vi "Test_EndOfList_ReturnLastItem.vi"(8 "error in (no error)":errorcluster, 11 "TestCase in":refnum<class "TestStringList.lvclass">) -> (0 "error out":errorcluster, 3 "TestCase out":refnum<class "TestStringList.lvclass">)   [LabVIEW 2015, in "StringList.lvlib" / "TestStringList.lvclass"]
uses:
  TestStringList.lvclass
  <vilib>/addons/_JKI Toolkits/VI Tester/TestCase.llb/TestCase.lvclass
  StringList.lvclass
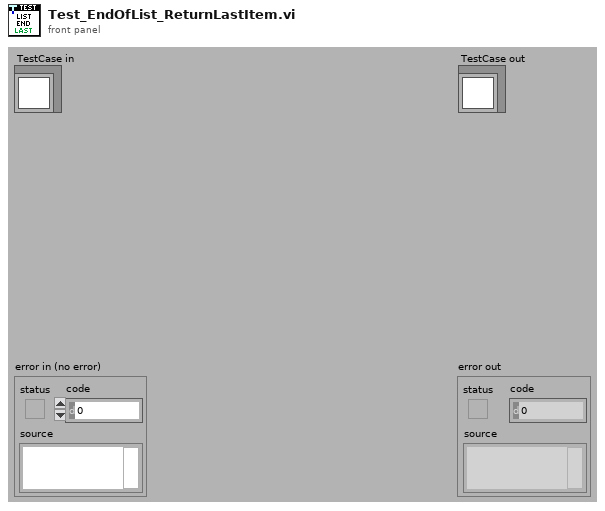
[diagram p1: front panel]
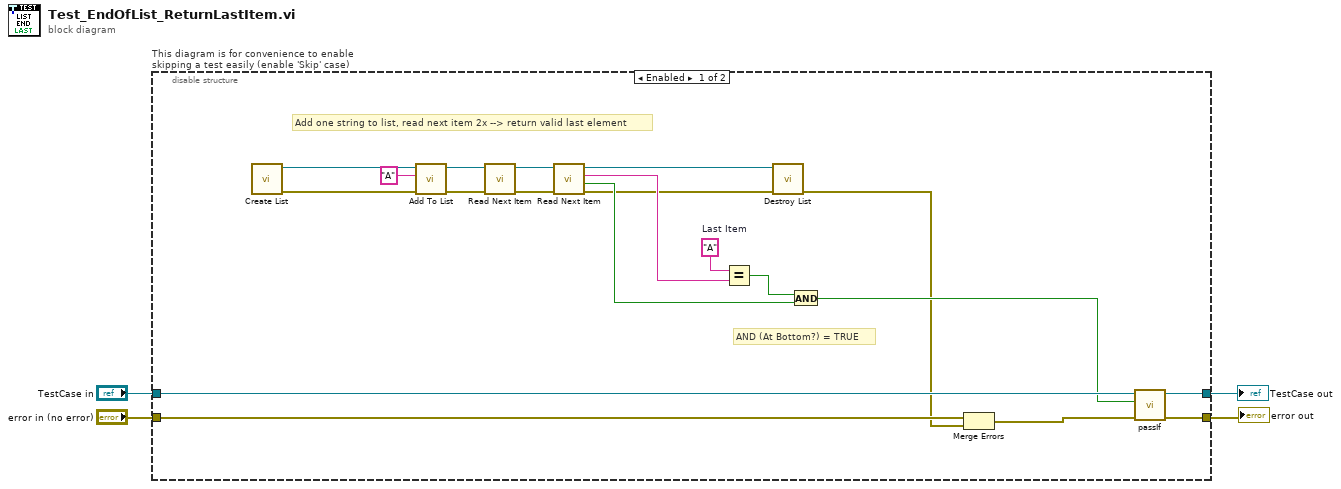
[diagram p0: block diagram]
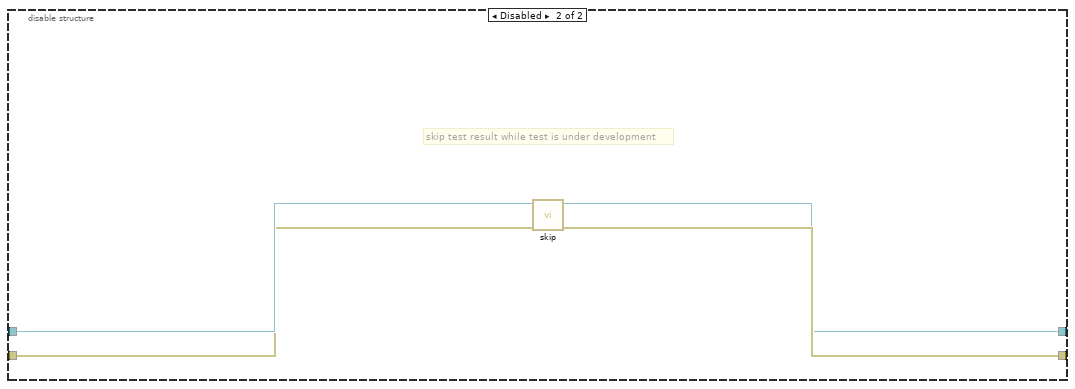
[diagram p2: hidden frame]
diagram:
  n1 = disable-structure "This diagram is for convenience to enable skipping a test easily (enable 'Skip' case)" shown="Enabled" {
    disable-tunnel: "TestCase in" -> [w24 w28]
    disable-tunnel: [w23 w26] -> w1
    disable-tunnel: [w22 w27] -> w3
    disable-tunnel: "error in (no error)" -> [w21 w25]
    frame Enabled {
      w15 = "A"  # Last Item
      # "AND (At Bottom?) = TRUE"
      # "Add one string to list, read next item 2x --> return valid last element"
      n2 = call "Create List.vi"() -> ("error out"=w10:errorcluster, "StringList Reference"=w17:refnum<data-value>)  [unwired: 10 in]
      n3 = call "Add To List.vi"("error in (no error)"=w10, "Item"="A", "StringList Reference"=w17) -> ("error out"=w9:errorcluster, "StringList Reference"=w20:refnum<data-value>)  [unwired: 7 in]
      n4 = call "Read Next Item.vi"("error in (no error)"=w9, "StringList Reference"=w20) -> ("error out"=w8:errorcluster, "StringList Reference"=w18:refnum<data-value>)  [unwired: 6 in, 2 out]
      n5 = call "Read Next Item.vi"("error in (no error)"=w8, "StringList Reference"=w18) -> ("error out"=w7:errorcluster, "At Bottom?"=w14:bool, "Item"=w16:string, "StringList Reference"=w11:refnum<data-value>)  [unwired: 6 in]
      n6 = Equal?(x=w15, y=w16) -> (x = y?=w13:bool)
      n7 = call "Destroy List.vi"("error in (no error)"=w7, "StringList Reference"=w11) -> ("error out"=w5:errorcluster)  [unwired: 8 in, 1 out]
      n8 = And(x=w13, y=w14) -> (x .and. y?=w12:bool)
      n9 = Merge Errors(w21, w5) -> (w6:errorcluster)
      n10 = call-dynamic "passIf.vi"("error in (no error)"=w6, "pass"=w12, "TestCase in"=w24) -> ("error out"=w22:errorcluster, "TestCase out"=w23:refnum<class "TestStringList.lvclass">)  [unwired: 7 in]
    }
    frame Disabled {
      # "skip test result while test is under development"
      n11 = call <vilib>:"skip.vi"("error in (no error)"=w25, "TestCase in"=w28) -> ("error out"=w27:errorcluster, "TestCase out"=w26:refnum<class "TestStringList.lvclass">)  [unwired: 8 in]
    }
  }
  "error out" <- w3
  "TestCase out" <- w1
